vi "Test ALL.vi"   [LabVIEW 2013]
uses:
  <vilib>/addons/_JKI Toolkits/Caraya/classes/Test/Test.lvclass
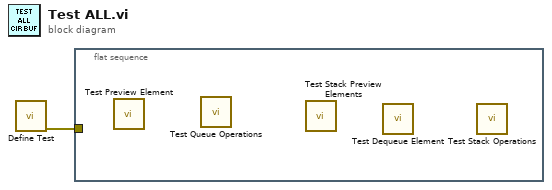
[diagram p0: block diagram]
diagram:
  n1 = call <vilib>:"Define Test.vi"() -> ("error out"=w1:errorcluster)  [unwired: 10 in, 1 out]
  n2 = flat-sequence {
    tunnel: w1 -> [_]
    frame #0 {
      n3 = call "Test Preview Element.vi"() -> ()  [unwired: 12 in]
      n4 = call "Test Queue Operations.vi"() -> ()  [unwired: 12 in]
      n5 = call "Test Stack Preview Elements.vi"() -> ()  [unwired: 12 in]
      n6 = call "Test Dequeue Element.vi"() -> ()  [unwired: 12 in]
      n7 = call "Test Stack Operations.vi"() -> ()  [unwired: 12 in]
    }
  }
